vi "simulator.vi"() -> ()   [LabVIEW 2012]
uses:
  gds_hw_config.lvlib
panel:
  out "error out":errorcluster
  out "BER":dbl
  out "Error (static)":dbl
  out "Estimated Offset":i32
  out "Delay":dbl
  out "Freq. Offset":dbl
  out "SNR (dB)":dbl
  in  "RX Parameters":T1 {"RX Sample Rate" items=["4M"]}
  in  "TX Parameters":T2 {"TX Sample Rate" items=["4M"]}
  in  "TX/RX Shared Parameters":T3
  in  "Channel Model Parameters":T4
  in  "RX Graphs":T5(tab)
  out "Received IQ Graph":cluster{dbl[], dbl[]}(graph) caption="IQ Graph"
  out "Received Constellation Graph":T6(graph) caption="Constellation Graph"
  out "Received Eye Diagram":cluster{"t0":dbl, "dt":dbl, "Y":dbl[]}[](graph) caption="Eye Diagram"
  out "Received Q":waveform(dbl)(graph)
  out "Received I":waveform(dbl)(graph)
  out "Received Phase":dbl[](graph)
  out "Received Magnitude":dbl[](graph)
  out "Received PSD":dbl[](graph)
  in  "TX Graphs":T7(tab)
  out "Transmitted IQ Graph":cluster{dbl[], dbl[]}(graph) caption="IQ Graph"
  out "Transmitted Constellation Graph":T6(graph) caption="Constellation Graph"
  out "Transmitted Eye Diagram":cluster{"t0":dbl, "dt":dbl, "Y":dbl[]}[](graph) caption="Eye Diagram"
  out "Transmitted Q":dbl[](graph)
  out "Transmitted I":dbl[](graph)
  out "Transmitted Phase":dbl[](graph)
  out "Transmitted Magnitude":dbl[](graph)
  out "Transmitted PSD":dbl[](graph)
  # "Measured Impairments"
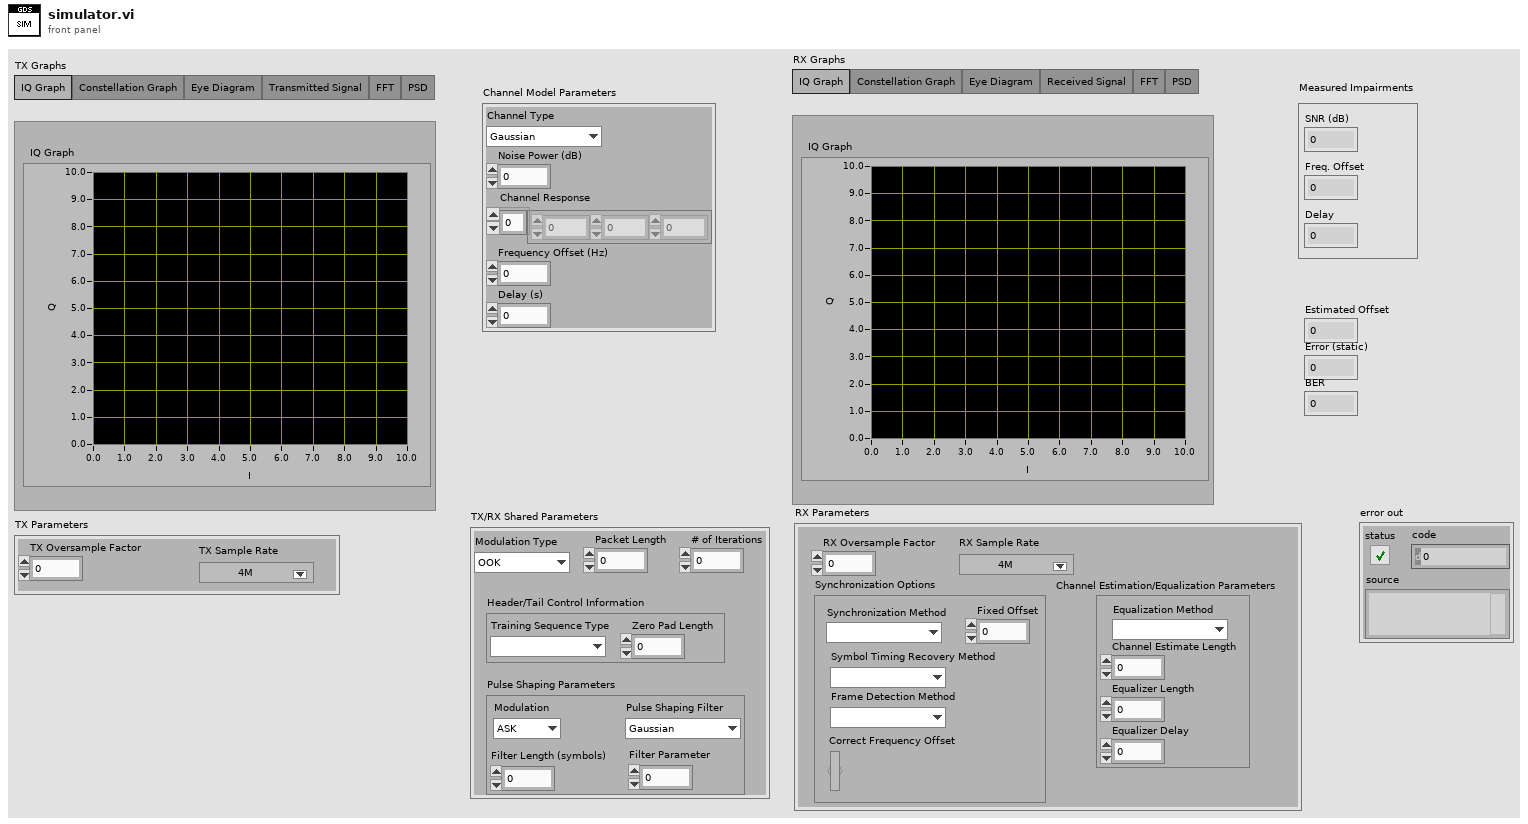
[diagram p1: front panel]
types:
  T1 = cluster{"RX Oversample Factor":dbl, "RX Sample Rate":u16, "Synchronization Options":cluster{"Synchronization Method":enum16{""}, "Symbol Timing Recovery Method ":enum16{""}, "Fixed Offset":dbl, "Frame Detection Method":enum16{""}, "Correct Frequency Offset":bool}, "Channel Estimation/Equalization Parameters":cluster{"Equalization Method":enum16{""}, "Channel Estimate Length":dbl, "Equalizer Length":dbl, "Equalizer Delay":dbl}}
  T2 = cluster{"TX Oversample Factor":dbl, "TX Sample Rate":u16}
  T3 = cluster{"Modulation Type":enum16{"OOK", "FSK"}, "Packet Length":dbl, "# of Iterations":u16, "Pulse Shaping Parameters":cluster{"Modulation":enum16{"ASK", "FSK", "PSK", "QAM", "MSK", "PAM"}, "Pulse Shaping Filter":enum16{"Gaussian"}, "Filter Length (symbols)":dbl, "Filter Parameter":dbl}, "Header/Tail Control Information":cluster{"Training Sequence Type":enum16{""}, "Zero Pad Length":dbl}}
  T4 = cluster{"Channel Type":enum16{"Gaussian", "ISI"}, "Noise Power (dB)":dbl, "Channel Response":cdb[], "Frequency Offset (Hz)":dbl, "Delay (s)":dbl}
  T5 = enum32{"IQ Graph", "Constellation Graph", "Eye Diagram", "Received Signal", "FFT", "PSD"}
  T6 = cluster{"Decimated Array":dbl[], "Decimated Array":dbl[]}[]
  T7 = enum32{"IQ Graph", "Constellation Graph", "Eye Diagram", "Transmitted Signal", "FFT", "PSD"}
  T8 = cluster{"TX Parameters":cluster{"TX Oversample Factor":dbl, "TX Sample Rate":u16}, "TX/RX Shared Parameters":cluster{"Modulation Type":enum16{"OOK", "FSK"}, "Packet Length":dbl, "# of Iterations":u16, "Pulse Shaping Parameters":cluster{"Modulation":enum16{"ASK", "FSK", "PSK", "QAM", "MSK", "PAM"}, "Pulse Shaping Filter":enum16{"Gaussian"}, "Filter Length (symbols)":dbl, "Filter Parameter":dbl}, "Header/Tail Control Information":cluster{"Training Sequence Type":enum16{""}, "Zero Pad Length":dbl}}}
  T9 = cluster{"RX Parameters":cluster{"RX Oversample Factor":dbl, "RX Sample Rate":u16, "Synchronization Options":cluster{"Synchronization Method":enum16{""}, "Symbol Timing Recovery Method ":enum16{""}, "Fixed Offset":dbl, "Frame Detection Method":enum16{""}, "Correct Frequency Offset":bool}, "Channel Estimation/Equalization Parameters":cluster{"Equalization Method":enum16{""}, "Channel Estimate Length":dbl, "Equalizer Length":dbl, "Equalizer Delay":dbl}}, "TX/RX Shared Parameters":cluster{"Modulation Type":enum16{"OOK", "FSK"}, "Packet Length":dbl, "# of Iterations":u16, "Pulse Shaping Parameters":cluster{"Modulation":enum16{"ASK", "FSK", "PSK", "QAM", "MSK", "PAM"}, "Pulse Shaping Filter":enum16{"Gaussian"}, "Filter Length (symbols)":dbl, "Filter Parameter":dbl}, "Header/Tail Control Information":cluster{"Training Sequence Type":enum16{""}, "Zero Pad Length":dbl}}}
  T10 = cluster{"SNR(dB)":dbl, "channel estimate":cdb[], "freq. offset":dbl, "delay":dbl}
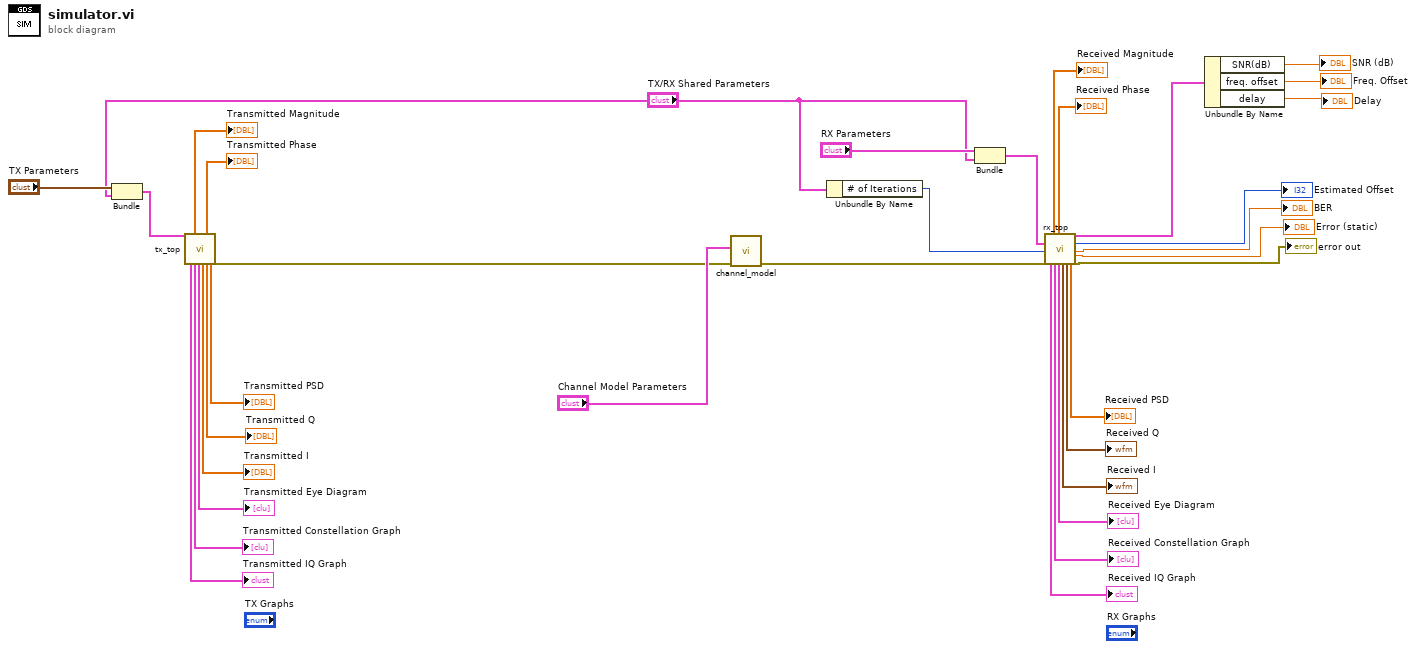
[diagram p0: block diagram]
diagram:
  n1 = Bundle("TX Parameters"="TX Parameters", "TX/RX Shared Parameters"="TX/RX Shared Parameters") -> (w29:T8)  [unwired: 1 in]
  n2 = call "tx_top.vi"("Modulation Parameters"=w29) -> ("Transmitted IQ Graph"=→"Transmitted IQ Graph":cluster{dbl[], dbl[]}, "Transmitted Magnitude"=→"Transmitted Magnitude":dbl[], "Transmitted Constellation Graph"=→"Transmitted Constellation Graph":T6, "Transmitted Eye Diagram"=→"Transmitted Eye Diagram":cluster{"t0":dbl, "dt":dbl, "Y":dbl[]}[], "Transmitted I"=→"Transmitted I":dbl[], "Transmitted Phase"=→"Transmitted Phase":dbl[], "Transmitted Q"=→"Transmitted Q":dbl[], "Transmitted PSD"=→"Transmitted PSD":dbl[], "error out"=w20:errorcluster)  [unwired: 17 in, 1 out]
  n3 = call "channel_model.vi"("error in (no error)"=w20, "Channel Model Parameters"="Channel Model Parameters") -> ("error out"=w19:errorcluster)  [unwired: 9 in]
  n4 = Unbundle By Name("TX/RX Shared Parameters") -> ("# of Iterations"=w17:u16)
  n5 = Bundle("RX Parameters"="RX Parameters", "TX/RX Shared Parameters"="TX/RX Shared Parameters") -> (w30:T9)  [unwired: 1 in]
  n6 = call "rx_top.vi"("Modulation Parameters"=w30, "# of Receive Iterations"=w17, "error in"=w19) -> ("Received IQ Graph"=→"Received IQ Graph":cluster{dbl[], dbl[]}, "Received Magnitude"=→"Received Magnitude":dbl[], "Received Constellation Graph"=→"Received Constellation Graph":T6, "Received Phase"=→"Received Phase":dbl[], "Received Eye Diagram"=→"Received Eye Diagram":cluster{"t0":dbl, "dt":dbl, "Y":dbl[]}[], "Received I"=→"Received I":waveform(dbl), "Received Q"=→"Received Q":waveform(dbl), "Received Power Spectrum Density"=→"Received PSD":dbl[], "Measured channel impairements"=w8:T10, "offset"=→"Estimated Offset":i32, "bit-error rate"=→"BER":dbl, "average \nbit-error rate"=→"Error (static)":dbl, "error out"=→"error out":errorcluster)  [unwired: 6 in, 6 out]
  n7 = Unbundle By Name(w8) -> ("SNR(dB)"=→"SNR (dB)":dbl, "freq. offset"=→"Freq. Offset":dbl, "delay"=→"Delay":dbl)
